vi "BL Get Channel.vi"() -> (2 "Other Channel Name":string, 3 "Channel Name":string)   [LabVIEW 2019]
uses:
  Globals.vi
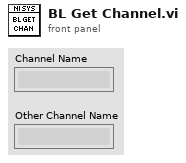
[diagram p1: front panel]
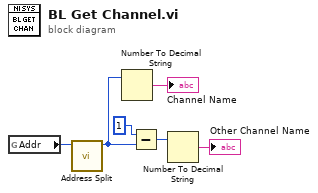
[diagram p0: block diagram]
diagram:
  n1 = global read "Globals.vi" "Addr"() -> (w1:u16)
  n2 = call "Address Split.vi"("address"=w1) -> ("sl_ext_sel"=w2:u32)  [unwired: 7 in, 3 out]
  n3 = Number To Decimal String(number=w2) -> (decimal integer string=→"Channel Name":string)  [unwired: 1 in]
  n4 = Subtract(x=u32 1, y=w2) -> (x-y=w4:u32)
  n5 = Number To Decimal String(number=w4) -> (decimal integer string=→"Other Channel Name":string)  [unwired: 1 in]
